vi "Op-Graphics-Scaling.vi"(8 "error in (no error)":errorcluster, 9 "operation":i32(slide) max=4 scale=0.0..4.0, 11 "VISA session":refnum<visa-resource-name>) -> (0 "error out":errorcluster, 3 "VISA resource name out":refnum<visa-resource-name>)   [LabVIEW 2016, in "Agilent 415X Series.lvlib"]
doc: "This VI scales the curve(s) displayed in GRAPHICS display mode. If the current display mode is LIST, it will be switched to GRAPHICS after this VI is executed."
uses:
  Agilent 415X Series.lvlib
panel:
  # "This VI will change the display mode to GRAPHICS"
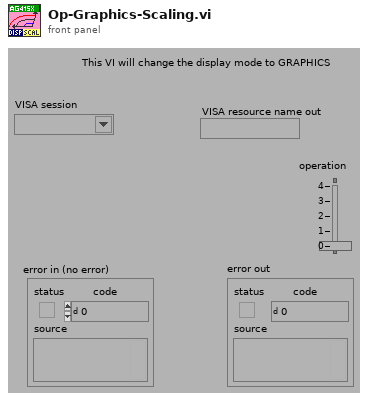
[diagram p1: front panel]
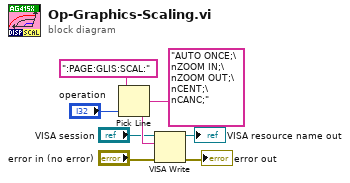
[diagram p0: block diagram]
diagram:
  n1 = Pick Line(string ("")=":PAGE:GLIS:SCAL:", multi-line string="AUTO ONCE;\nZOOM IN;\nZOOM OUT;\nCENT;\nCANC;", line index="operation") -> (output string=w5:string)
  n2 = VISA Write(VISA resource name="VISA session", write buffer=w5, error in (no error)="error in (no error)") -> (VISA resource name out=→"VISA resource name out":refnum<visa-resource-name>, error out=→"error out":errorcluster)  [unwired: 1 out]
